vi "Passwort SystemLevel.vi"(9 "reset":bool, 10 "Passworte gelesen":T1, 11 "Default Passworte":T1) -> (3 "Passworte":T1)   [LabVIEW 2020, in "Passwort.lvlib"]
uses:
  Passwort.lvlib
  Passwort Array.ctl
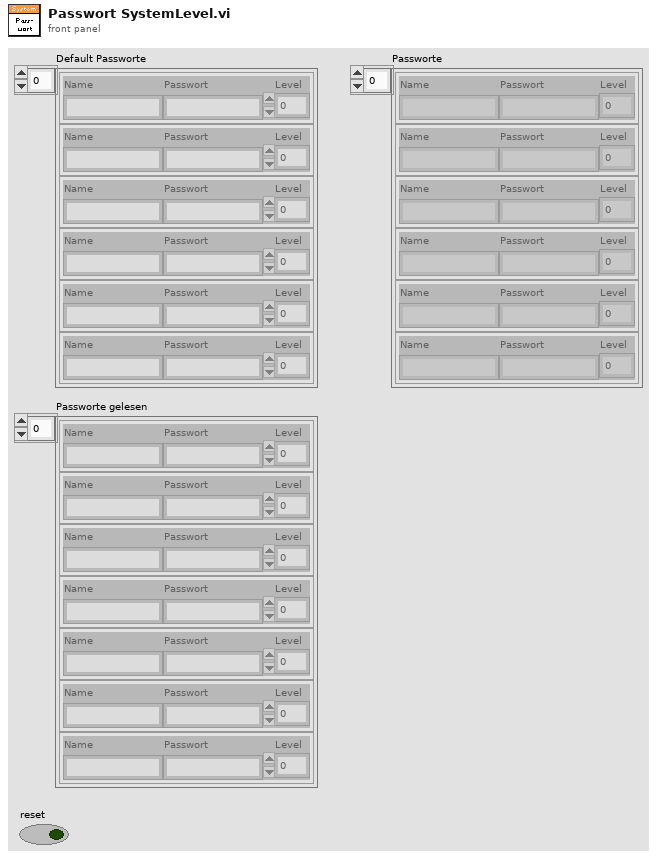
[diagram p1: front panel]
types:
  T1 = typedef "Passwort.lvlib/Passwort Array.ctl" = cluster{"Name":string, "Passwort":string, "Level":i16}[]
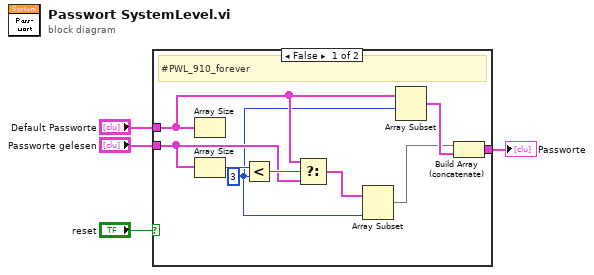
[diagram p0: block diagram]
diagram:
  n1 = case shown="False" "reset" {
    tunnel: [w12 w14] -> w4
    tunnel: "Default Passworte" -> [w10 w14]
    tunnel: "Passworte gelesen" -> [w9 _]
    frame False {
      w6 = 3 ("y")
      # "#PWL_910_forever"
      n2 = Array Size(array=w10) -> ()  [unwired: 1 out]
      n3 = Array Size(array=w9) -> (size(s)=w13:i32)
      n4 = Less?(x=w13, y=w6) -> (x < y?=w11:bool)
      n5 = Select(t=w10, s=w11, f=w9) -> (s? t:f=w7:T1)
      n6 = Array Subset(array=w7, length=w6) -> (w5:T1)  [unwired: 1 in]
      n7 = Array Subset(array=w10, index=w6) -> (w8:T1)  [unwired: 1 in]
      n8 = Build Array (concatenate)(w5, w8) -> (w12:T1)
    }
    frame True {
    }
  }
  "Passworte" <- w4
